vi "Random Series.vi"() -> ()   [LabVIEW 2023]
doc: "This VI demonstrates the use of the Accumulator Tag channel by simulating multiple randomseries with different values."
uses:
  <extravilib>/ChannelInstances/Tag-bool/Read With Abort.vi
  <extravilib>/ChannelInstances/Accumulator Tag-dbl/Write With Abort.vi
  <extravilib>/ChannelInstances/Accumulator Tag-dbl/Read With Abort.vi
  <extravilib>/ChannelInstances/Tag-bool/Write With Abort.vi
  <extravilib>/ChannelInstances/Accumulator Tag-dbl/Endpoint.vi
  <extravilib>/ChannelInstances/Accumulator Tag-dbl/EndpointRead.vi
  <extravilib>/ChannelInstances/Tag-bool/Instantiate.vi
  <extravilib>/ChannelInstances/Accumulator Tag-dbl/Instantiate.vi
  <extravilib>/ChannelInstances/Tag-bool/Endpoint.vi
  <extravilib>/ChannelInstances/Accumulator Tag-dbl/))Channel.vi
  <extravilib>/ChannelInstances/Tag-bool/EndpointRead.vi
  <extravilib>/ChannelInstances/Tag-bool.lvlib
  <extravilib>/ChannelInstances/Accumulator Tag-dbl.lvlib
panel:
  out "events":i32
  in  "Stop":bool
  in  "average":bool
  out "value":dbl format="$%.2f"
  # "Overview: Demonstrates the use of the Accumulator Tag channel simulating multiple random series with different values.\n\nInstructions:\nRun the VI.  Observe the total value and number of events each second.  Click the average switch to observe the average value per event during each second."
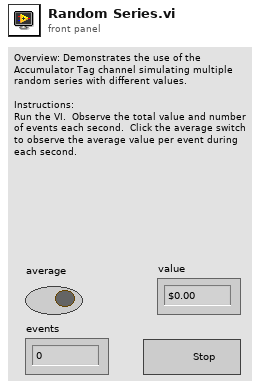
[diagram p1: front panel]
types:
  T1 = typedef "Tag-bool.lvlib/))Channel.ctl" = refnum<queue>
  T2 = typedef "Accumulator Tag-dbl.lvlib/))Channel.ctl" = refnum<queue>
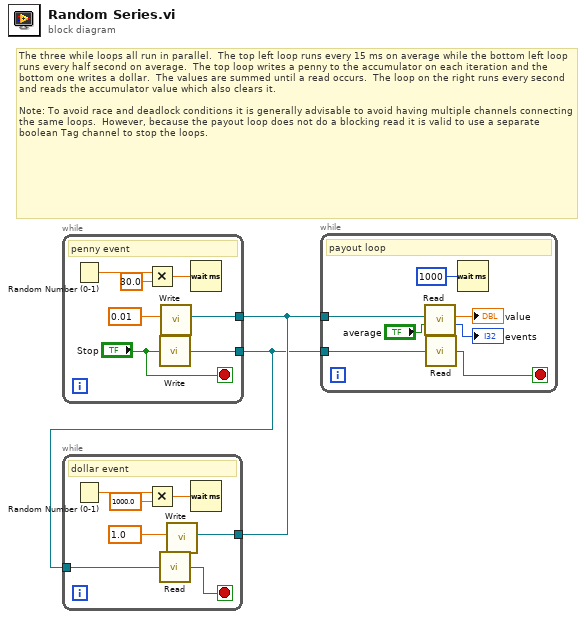
[diagram p0: block diagram]
diagram:
  # "The three while loops all run in parallel.  The top left loop runs every 15 ms on average while the bottom left loop runs every half second on average.  The top loop writes a penny to the accumulator on each iteration and the bottom one writes a dollar.  The values are summed until a read occurs.  The loop on the right runs every second and reads the accumulator value which also clears it.\n\nNote: To avoid race and deadlock conditions it is generally advisable to avoid having multiple channels connecting the same loops.  However, because the payout loop does not do a blocking read it is valid to use a separate boolean Tag channel to stop the loops."
  n1 = while {
    tunnel: w2 -> [w3]
    tunnel: [w5] -> w1
    stop <- "Stop" stop-if-true
    # "penny event"
    n2 = Random Number (0-1)() -> (number: 0 to 1=w9:dbl)
    n3 = Multiply(x=w9, y=30.0) -> (x*y=w7:dbl)
    n4 = call <extravilib>:"Write.vi"("element"="Stop") -> ("channel"=w5:T1)  [unwired: 1 out]
    n5 = call <extravilib>:"Write.vi"("element"=0.01) -> ("channel"=w3:T2)  [unwired: 10 in]
    n6 = Wait (ms)(milliseconds to wait=w7) -> ()  [unwired: 1 out]
  }
  n7 = while {
    tunnel: [w10] -> w2
    tunnel: w1 -> [w12]
    stop <- w13 stop-if-true
    # "dollar event"
    n8 = Random Number (0-1)() -> (number: 0 to 1=w16:dbl)
    n9 = Multiply(x=w16, y=1000.0) -> (x*y=w14:dbl)
    n10 = call <extravilib>:"Read.vi"("channel"=w12) -> ("element"=w13:bool)  [unwired: 1 in, 1 out]
    n11 = call <extravilib>:"Write.vi"("element"=1.0) -> ("channel"=w10:T2)  [unwired: 10 in]
    n12 = Wait (ms)(milliseconds to wait=w14) -> ()  [unwired: 1 out]
  }
  n13 = while {
    tunnel: w2 -> [w20]
    tunnel: w1 -> [w22]
    stop <- w21 stop-if-true
    # "payout loop"
    n14 = call <extravilib>:"Read.vi"("average (F)"="average", "channel"=w20) -> ("count"=→"events":i32, "element"=→"value":dbl)  [unwired: 8 in]
    n15 = call <extravilib>:"Read.vi"("channel"=w22) -> ("element"=w21:bool)  [unwired: 1 in, 1 out]
    n16 = Wait (ms)(milliseconds to wait=u32 1000) -> ()  [unwired: 1 out]
  }
